vi "G# - InterfaceDemo.vi"() -> ()   [LabVIEW 2020]
doc: "G# Interface Implementation\nThis examples demonstrates how to use the G#Interface. The interface concept is an alternative design principle to multiple inheritance (just as in C# and Java). Classes that are not related can implement the same interface and the reference of the interface could be treated just as they are from the same class.\n\nBy using the G# Debugger found in Tools->G# Debugger a text log can be followed showing how the objects were created and destroyed."
uses:
  IMyInterface1_interface/IMyInterface1.lvclass
  IMyInterface2_interface/IMyInterface2.lvclass
  MyClass2_class/MyClass2.lvclass
  C:/ProjectGSharpDevelopment_2020-3/gsharp/VIPM/Files/examples/Object-Oriented G# Development/Interface/IMyInterface1_interface/IMyInterface1.lvclass
  MyClass1_class/MyClass1.lvclass
  vi.lib/addons/_AddQ/G#Object/G#Object.lvclass
panel:
  out "MyClass2 is NOT instance of IMyInterface2":bool
  out "MyClass1 is instance of IMyInterface2":bool
  out "# of objects killed":i32
  out "OK":bool
  in  "error in (no error)":errorcluster
  out "MyClass2 is instance of IMyInterface1":bool
  out "MyClass1 is instance of IMyInterface1":bool
  out "error out":errorcluster
  out "Class Name":string[](array[string])
  # "G# Interface Implementation native Interface in LV2020\nThis examples demonstrates how to use the native interface in LV2020 with G#. Classes that are not related can implement the same interface\nand the reference of the interface could be treated just as they are from the same class.\n\nBy using the G# Debugger found in Tools->G# Debugger a text log can be followed showing how the objects were created and destroyed."
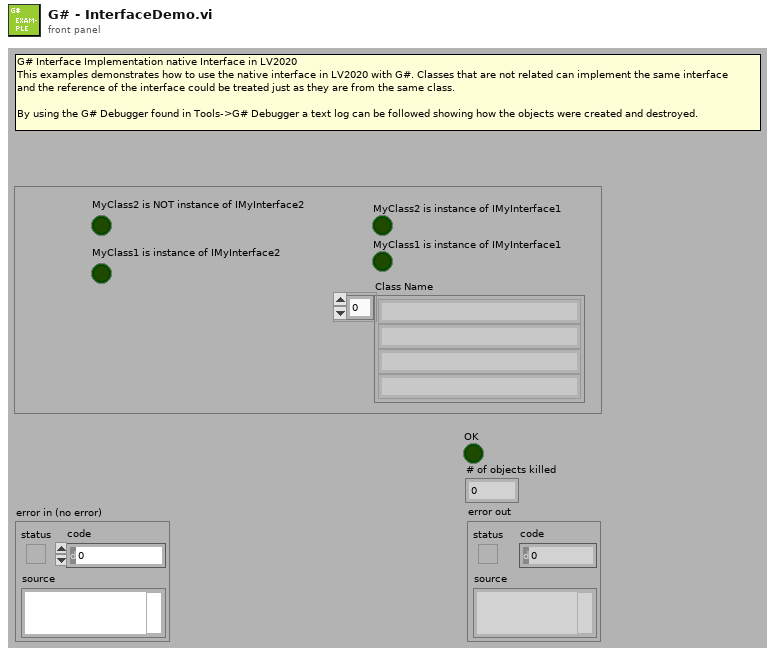
[diagram p1: front panel]
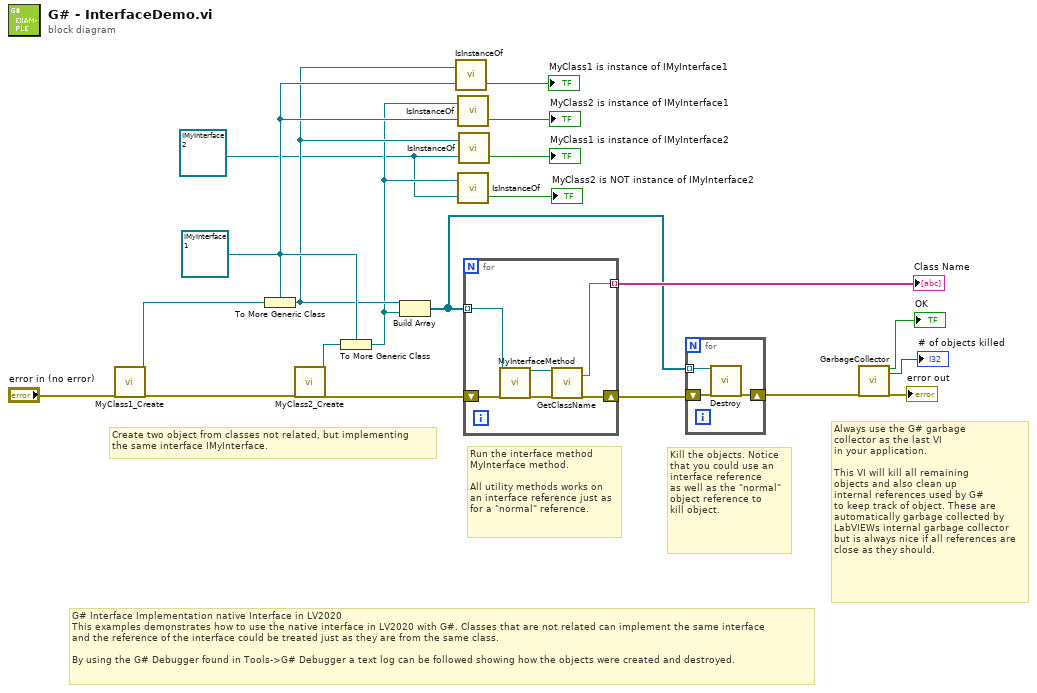
[diagram p0: block diagram]
diagram:
  w4 = refnum<class "IMyInterface2.lvclass"> refnum ("IMyInterface2")
  w8 = refnum<class "IMyInterface1.lvclass"> refnum ("IMyInterface3")
  # "G# Interface Implementation native Interface in LV2020\nThis examples demonstrates how to use the native interface in LV2020 with G#. Classes that are not related can implement the same interface\nand the reference of the interface could be treated just as they are from the same class.\n\nBy using the G# Debugger found in Tools->G# Debugger a text log can be followed showing how the objects were created and destroyed."
  # "Always use the G# garbage\ncollector as the last VI\nin your application.\n\nThis VI will kill all remaining\nobjects and also clean up\ninternal references used by G#\nto keep track of object. These are\nautomatically garbage collected by\nLabVIEWs internal garbage collector\nbut is always nice if all references are\nclose as they should."
  # "Kill the objects. Notice\nthat you could use an\ninterface reference\nas well as the \"normal\"\nobject reference to\nkill object."
  # "Run the interface method\nMyInterface method.\n\nAll utility methods works on\nan interface reference just as\nfor a \"normal\" reference."
  # "Create two object from classes not related, but implementing\nthe same interface IMyInterface."
  n1 = call "MyClass1_Create.vi"("error in (no error)"="error in (no error)") -> ("reference out"=w2:refnum<class "MyClass1.lvclass">, "error out"=w13:errorcluster)  [unwired: 17 in]
  n2 = To More Generic Class(target class=w8, reference=w2) -> (generic class reference=w7:refnum<class "IMyInterface1.lvclass">)
  n3 = call "MyClass2_Create.vi"("error in (no error)"=w13) -> ("reference out"=w1:refnum<class "MyClass2.lvclass">, "error out"=w12:errorcluster)  [unwired: 17 in]
  n4 = To More Generic Class(target class=w8, reference=w1) -> (generic class reference=w5:refnum<class "IMyInterface1.lvclass">)
  n5 = Build Array(w7, w5) -> (w11:refnum<class "IMyInterface1.lvclass">[])
  n6 = call-dynamic "IsInstanceOf.vi"("is object instance of"=w8, "reference in"=w7) -> ("is instance of"=→"MyClass1 is instance of IMyInterface1":bool)  [unwired: 1 out]
  n7 = call-dynamic "IsInstanceOf.vi"("is object instance of"=w8, "reference in"=w5) -> ("is instance of"=→"MyClass2 is instance of IMyInterface1":bool)  [unwired: 1 out]
  n8 = call-dynamic "IsInstanceOf.vi"("is object instance of"=w4, "reference in"=w5) -> ("is instance of"=→"MyClass2 is NOT instance of IMyInterface2":bool)  [unwired: 1 out]
  n9 = call-dynamic "IsInstanceOf.vi"("is object instance of"=w4, "reference in"=w7) -> ("is instance of"=→"MyClass1 is instance of IMyInterface2":bool)  [unwired: 1 out]
  n10 = for {
    shift-right: [w24] -> w19
    shift-left: w12 -> [w26]
    tunnel: w11 -> [w25] mode=indexing
    tunnel: [w23] -> w18 mode=indexing
    n11 = call-dynamic "MyInterfaceMethod.vi"("reference in"=w25, "error in (no error)"=w26) -> ("reference out"=w22:refnum<class "IMyInterface1.lvclass">, "error out"=w21:errorcluster)  [unwired: 16 in]
    n12 = call-dynamic "GetClassName.vi"("reference in"=w22, "error in (no error)"=w21) -> ("class name"=w23:string, "error out"=w24:errorcluster)  [unwired: 13 in, 3 out]
  }
  "Class Name" <- w18
  n13 = for {
    shift-right: [w28] -> w17
    shift-left: w19 -> [w29]
    tunnel: w11 -> [w27] mode=indexing
    n14 = call-dynamic "Destroy.vi"("reference in"=w27, "error in (no error)"=w29) -> ("error out"=w28:errorcluster)  [unwired: 16 in, 1 out]
  }
  n15 = call "GarbageCollector.vi"("error in (no error)"=w17) -> ("OK"=→"OK":bool, "# of objects killed"=→"# of objects killed":i32, "error out"=→"error out":errorcluster)  [unwired: 16 in]
